vi "ClassInheritanceEditor_Interface.vi"(9 "EventsIn":T1, 10 "Events":T2) -> ()   [LabVIEW 2014, in "ClassInheritanceEditor.lvlib" / "ClassInheritanceEditor.lvclass"]
uses:
  ClassInheritanceEditor.lvclass
  Framework/_Plugins/_LVCMPlugin/GCMPlugin_EventsOut.ctl
  Framework/_Plugins/_LVCMPlugin/GCMPlugin_EventsIn.ctl
  State.ctl
  Framework/_Plugins/GCMPlugin/GCMPlugin.lvclass
panel:
  in  "InheritanceTree":string(tree)
  in  "Current parent":string
  in  "New parent":string
  in  "ChangeParent":bool
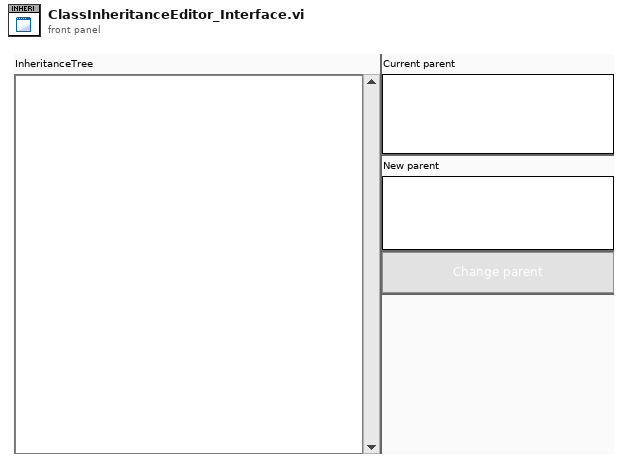
[diagram p1: front panel]
types:
  T1 = typedef "GCMPlugin.lvclass/GCMPlugin_EventsIn.ctl" = cluster{"Stop":refnum<user-event>, "ItemSelected":refnum<user-event>, "ItemDeselected":refnum<user-event>, "PluginActivated":refnum<user-event>, "PluginDeactivated":refnum<user-event>}
  T2 = typedef "GCMPlugin.lvclass/GCMPlugin_EventsOut.ctl" = cluster{"ItemEdited":refnum<user-event>}
  T3 = typedef "ClassInheritanceEditor.lvlib/ClassInheritanceEditor.lvclass/State.ctl" = enum16{"Initialize", "WaitForEvent", "Stop"}
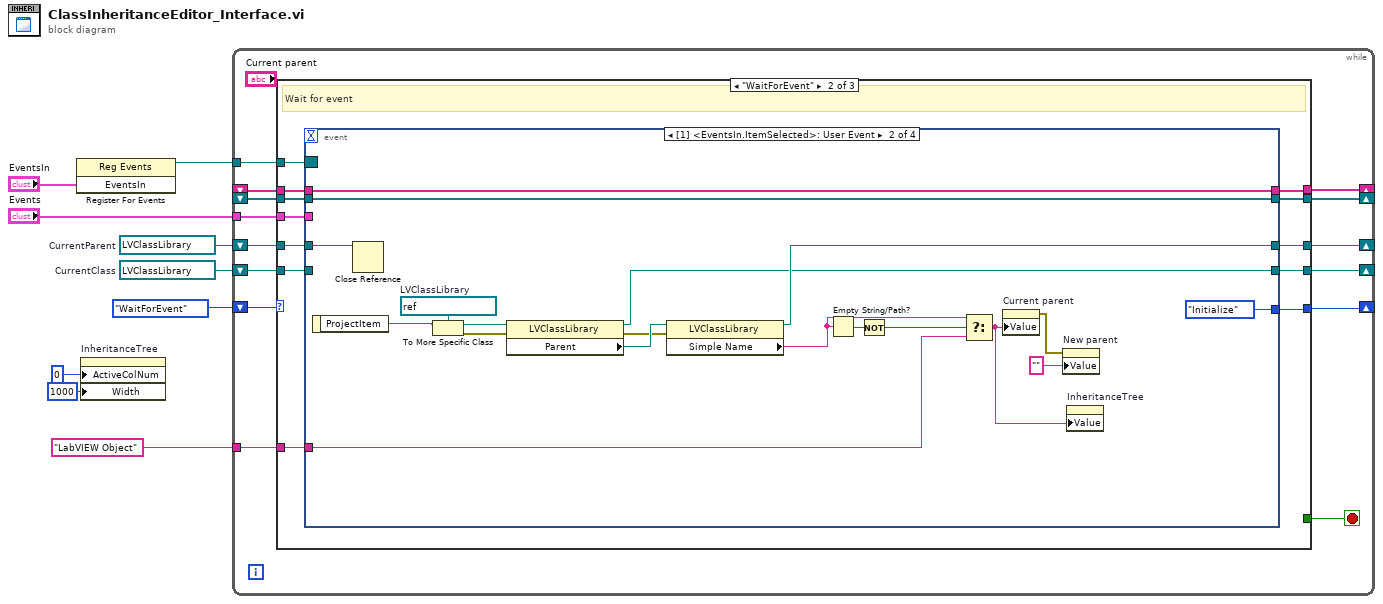
[diagram p0: block diagram]
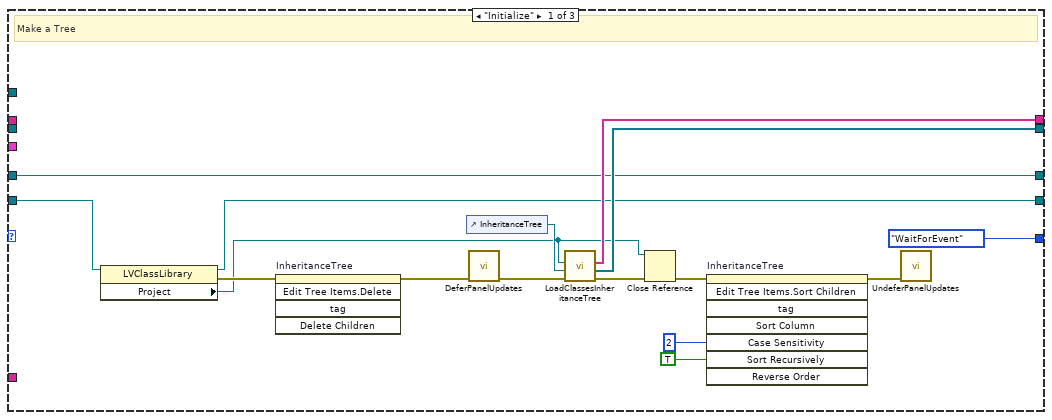
[diagram p2: hidden frame]
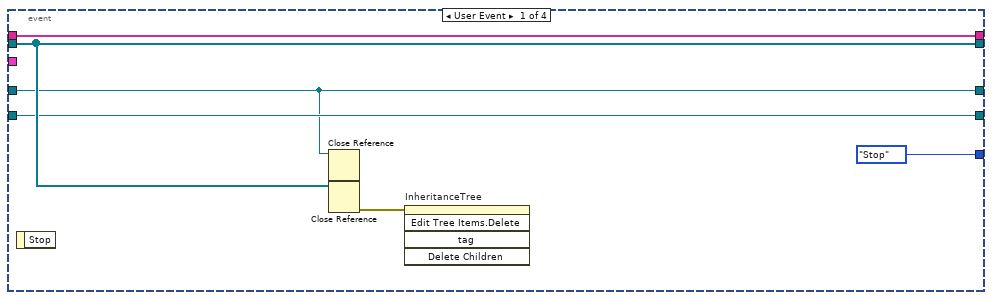
[diagram p3: hidden frame]
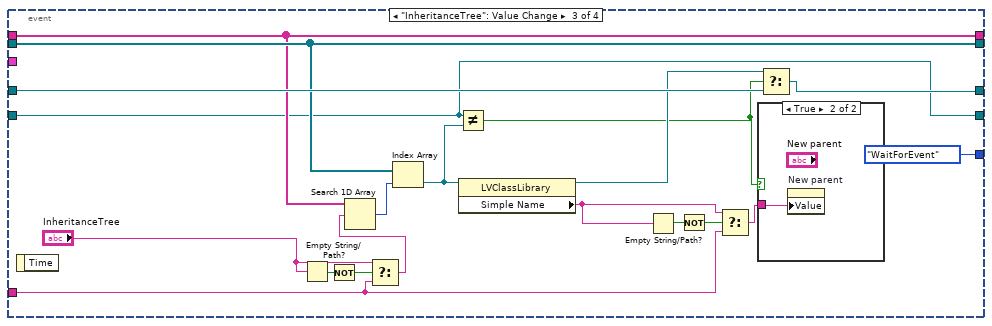
[diagram p4: hidden frame]
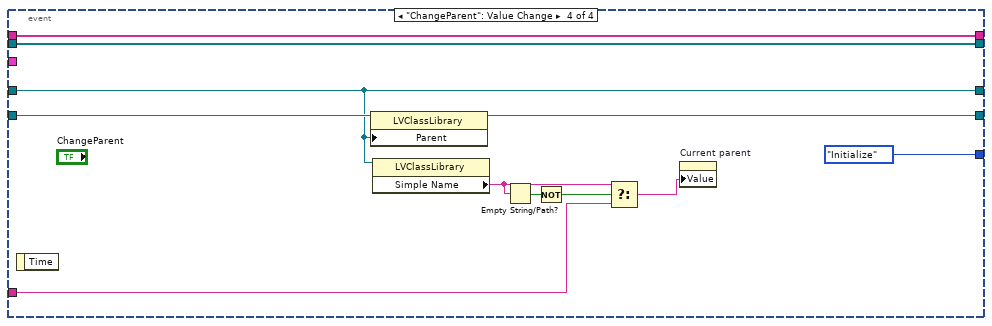
[diagram p6: hidden frame]
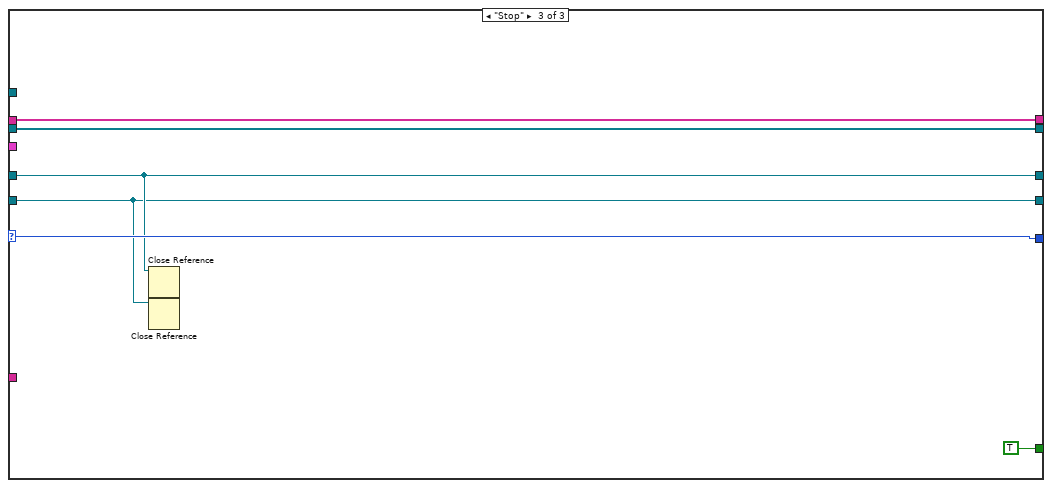
[diagram p7: hidden frame]
diagram:
  w3 = refnum<vi> refnum  # CurrentClass
  w4 = refnum<vi> refnum  # CurrentParent
  n1 = register-events("EventsIn") -> (reference out=w8:refnum<event-registration>)  [unwired: 2 in, 1 out]
  n2 = property on="InheritanceTree" class="Tree (strict)"("ActiveColNum"=0 ("Active Cell:Active Column Number"), "Width"=1000 ("Active Cell:Cell Size:Width")) -> ()  [unwired: 2 in, 2 out]
  n3 = while {
    tunnel: w8 -> [w23]
    tunnel: "Events" -> [w22]
    shift-right: [w16] -> _
    shift-left: w4 -> [w17]
    shift-right: [w12] -> _
    shift-left: State."WaitForEvent" ("State") -> [w15]
    shift-right: [w14] -> _
    shift-left: _ -> [w19]
    shift-right: [w13] -> _
    shift-left: _ -> [w18]
    tunnel: "LabVIEW Object" ("t") -> [w11]
    shift-right: [w10] -> _
    shift-left: w3 -> [w20]
    stop <- w21 stop-if-true
    n4 = case shown="\"WaitForEvent\"" w15 {
      selector: w15 -> [_ _ w113]
      tunnel: w23 -> [_ w51 _]
      tunnel: w22 -> [_ w50 _]
      tunnel: [_ _ TRUE ("Stop")] -> w21
      tunnel: w20 -> [w27 w49 w108]
      tunnel: w19 -> [_ w48 w112]
      tunnel: w18 -> [_ w47 w111]
      tunnel: w17 -> [w29 w46 w109]
      tunnel: [w29 w45 w109] -> w16
      tunnel: [w39 w43 w112] -> w14
      tunnel: [w38 w42 w111] -> w13
      tunnel: [State."WaitForEvent" w44 w113] -> w12
      tunnel: w11 -> [_ w41 _]
      tunnel: [w26 w40 w108] -> w10
      frame "Initialize" {
        # "Make a Tree"
        n5 = property class="LVClassLibrary"(reference=w27) -> (reference out=w26:refnum<vi>, error out=w28:errorcluster, "Project"=w24:refnum<vi>)  [unwired: 1 in]
        n6 = invoke on="InheritanceTree" class="Tree (strict)" method="Edit Tree Items.Delete"(error in=w28) -> (error out=w33:errorcluster)  [unwired: 4 in, 4 out]
        n7 = control-ref of="InheritanceTree"() -> (w31:refnum<vi>)
        n8 = call "DeferPanelUpdates.vi"("error in (no error)"=w33) -> ("error out"=w32:errorcluster)  [unwired: 10 in]
        n9 = call "LoadClassesInheritanceTree.vi"("error in (no error)"=w32, "TreeControl"=w31, "Project"=w24) -> ("error out"=w34:errorcluster, "Classes"=w38:refnum<vi>[], "ClassesNames"=w39:string[])  [unwired: 6 in]
        n10 = Close Reference(reference=w24, error in (no error)=w34) -> (error out=w25:errorcluster)
        n11 = invoke on="InheritanceTree" class="Tree (strict)" method="Edit Tree Items.Sort Children"(error in=w25, "Case Sensitivity"=2, "Sort Recursively"=TRUE ("Sort Recursively?")) -> (error out=w35:errorcluster)  [unwired: 5 in, 7 out]
        n12 = call "UndeferPanelUpdates.vi"("error in (no error)"=w35) -> ()  [unwired: 10 in, 1 out]
      }
      frame "WaitForEvent" {
        # "Wait for event"
        n13 = event shown="[1] <EventsIn.ItemSelected>: User Event" {
          selector: w51 -> [_ _ _ _]
          dyn-events: _ -> [_ _ _ _]
          timeout: _ -> [_ _ _ _]
          tunnel: w50 -> [_ _ _ _]
          tunnel: w49 -> [w53 _ w77 w107]
          tunnel: w48 -> [w54 w76 w83 w105]
          tunnel: w47 -> [w55 w75 w84 w104]
          tunnel: w46 -> [w52 w62 w93 w99]
          tunnel: [w52 w63 w90 w99] -> w45
          tunnel: [State."Stop" State."Initialize" State."WaitForEvent" State."Initialize"] -> w44
          tunnel: [w54 w76 w83 w105] -> w43
          tunnel: [w55 w75 w84 w104] -> w42
          tunnel: w41 -> [_ w59 w80 w98]
          tunnel: [w53 w61 w77 w97] -> w40
          event User Event {
            n14 = event-data() -> ()  [unwired: 1 in, 1 out]
            n15 = Close Reference(reference=w52) -> ()  [unwired: 1 in, 1 out]
            n16 = Close Reference(reference=w55) -> (error out=w57:errorcluster)  [unwired: 1 in]
            n17 = invoke on="InheritanceTree" class="Tree (strict)" method="Edit Tree Items.Delete"(error in=w57) -> ()  [unwired: 4 in, 5 out]
          }
          event User Event {
            w67 = refnum<vi> refnum  # LVClassLibrary
            n18 = event-data() -> ("ProjectItem"=w66:refnum<vi>)  [unwired: 1 in]
            n19 = Close Reference(reference=w62) -> ()  [unwired: 1 in, 1 out]
            n20 = To More Specific Class(target class=w67, reference=w66) -> (specific class reference=w68:refnum<vi>, error out=w64:errorcluster)  [unwired: 1 in]
            n21 = property class="LVClassLibrary"(reference=w68, error in=w64) -> (reference out=w61:refnum<vi>, error out=w65:errorcluster, "Parent"=w69:refnum<vi>)
            n22 = property class="LVClassLibrary"(reference=w69, error in=w65) -> (reference out=w63:refnum<vi>, "Simple Name"=w72:string)  [unwired: 1 out]
            n23 = Empty String/Path?(string/path=w72) -> (empty?=w71:bool)
            n24 = Not(x=w71) -> (.not. x?=w70:bool)
            n25 = Select(t=w72, s=w70, f=w59) -> (s? t:f=w58:string)
            n26 = property on="Current parent" class="Str"("Value"=w58) -> (error out=w73:errorcluster)  [unwired: 2 in, 1 out]
            n27 = property on="New parent" class="Str"(error in=w73, "Value"="" ("NewParent")) -> ()  [unwired: 1 in, 2 out]
            n28 = property on="InheritanceTree" class="Tree (strict)"("Value"=w58) -> ()  [unwired: 2 in, 2 out]
          }
          event "InheritanceTree": Value Change {
            n29 = event-data() -> ()  [unwired: 1 in, 1 out]
            n30 = Empty String/Path?(string/path="InheritanceTree") -> (empty?=w82:bool)
            n31 = Not(x=w82) -> (.not. x?=w81:bool)
            n32 = Select(t="InheritanceTree", s=w81, f=w80) -> (s? t:f=w78:string)
            n33 = Search 1D Array(1D array=w83, element=w78) -> (index of element=w95:i32)  [unwired: 1 in]
            n34 = Index Array(array=w84, index=w95) -> (element=w94:refnum<vi>)
            n35 = Not Equal?(x=w77, y=w94) -> (x != y?=w91:bool)
            n36 = property class="LVClassLibrary"(reference=w94) -> (reference out=w92:refnum<vi>, "Simple Name"=w86:string)  [unwired: 1 in, 1 out]
            n37 = Empty String/Path?(string/path=w86) -> (empty?=w88:bool)
            n38 = Not(x=w88) -> (.not. x?=w87:bool)
            n39 = Select(t=w86, s=w87, f=w80) -> (s? t:f=w89:string)
            n40 = case shown="True" w91 {
              tunnel: w89 -> [_ w96]
              frame False {
              }
              frame True {
                n41 = property on="New parent" class="Str"("Value"=w96) -> ()  [unwired: 2 in, 2 out]
              }
            }
            n42 = Select(t=w92, s=w91, f=w93) -> (s? t:f=w90:refnum<vi>)
          }
          event "ChangeParent": Value Change {
            n43 = event-data() -> ()  [unwired: 1 in, 1 out]
            n44 = property class="LVClassLibrary"(reference=w107, "Parent"=w99) -> (reference out=w97:refnum<vi>)  [unwired: 1 in, 1 out]
            n45 = property class="LVClassLibrary"(reference=w99) -> ("Simple Name"=w102:string)  [unwired: 1 in, 2 out]
            n46 = Empty String/Path?(string/path=w102) -> (empty?=w101:bool)
            n47 = Not(x=w101) -> (.not. x?=w100:bool)
            n48 = Select(t=w102, s=w100, f=w98) -> (s? t:f=w103:string)
            n49 = property on="Current parent" class="Str"("Value"=w103) -> ()  [unwired: 2 in, 2 out]
          }
        }
      }
      frame "Stop" {
        n50 = Close Reference(reference=w109) -> ()  [unwired: 1 in, 1 out]
        n51 = Close Reference(reference=w108) -> ()  [unwired: 1 in, 1 out]
      }
    }
  }
